vi "windows_folder_paths.vi"(8 "error in (no error)":errorcluster, 9 "Create Folder if not found? (F)":bool, 10 "Return non-default path?":enum32{"current path", "default path"}(ring), 11 "Folder Role":i32(ring)) -> (0 "error out":errorcluster {"code" format="%.0x"}, 1 "Description":string, 3 "System Folder Path":path)   [LabVIEW 2015]
doc: "This VI calls a Windows API function to retrieve the path of Windows System Folders that may vary with different installations of the operating system."
uses:
  shell32.dll
panel:
  # "These are CSIDL (constant special item ID list)\ncodes from the Windows API"
  # "The current folder may differ from the \ndefault if the user moved it or renamed it."
  # "Note:  CSIDL values are defined in Windows header file shlobj.h. \nFor a list of CSIDL constants, search Microsoft's web site for \"CSIDL\".\n\nThe function and constants used in this VI are supported on Win2000,\nWinXP, and Vista."
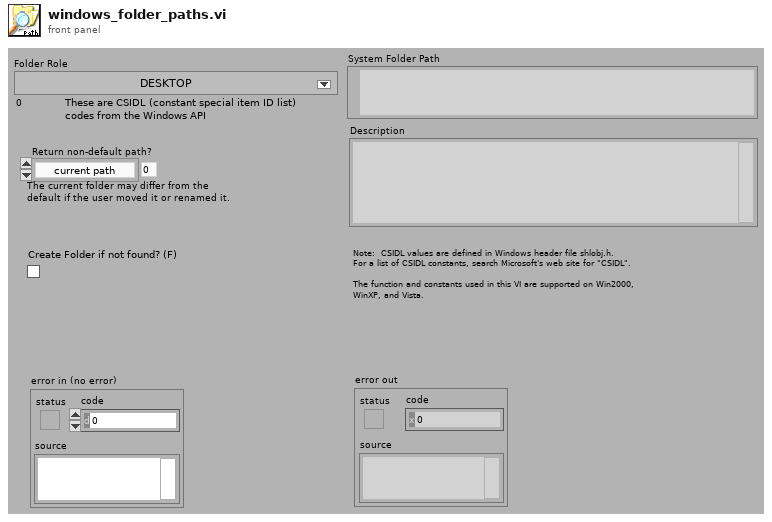
[diagram p1: front panel]
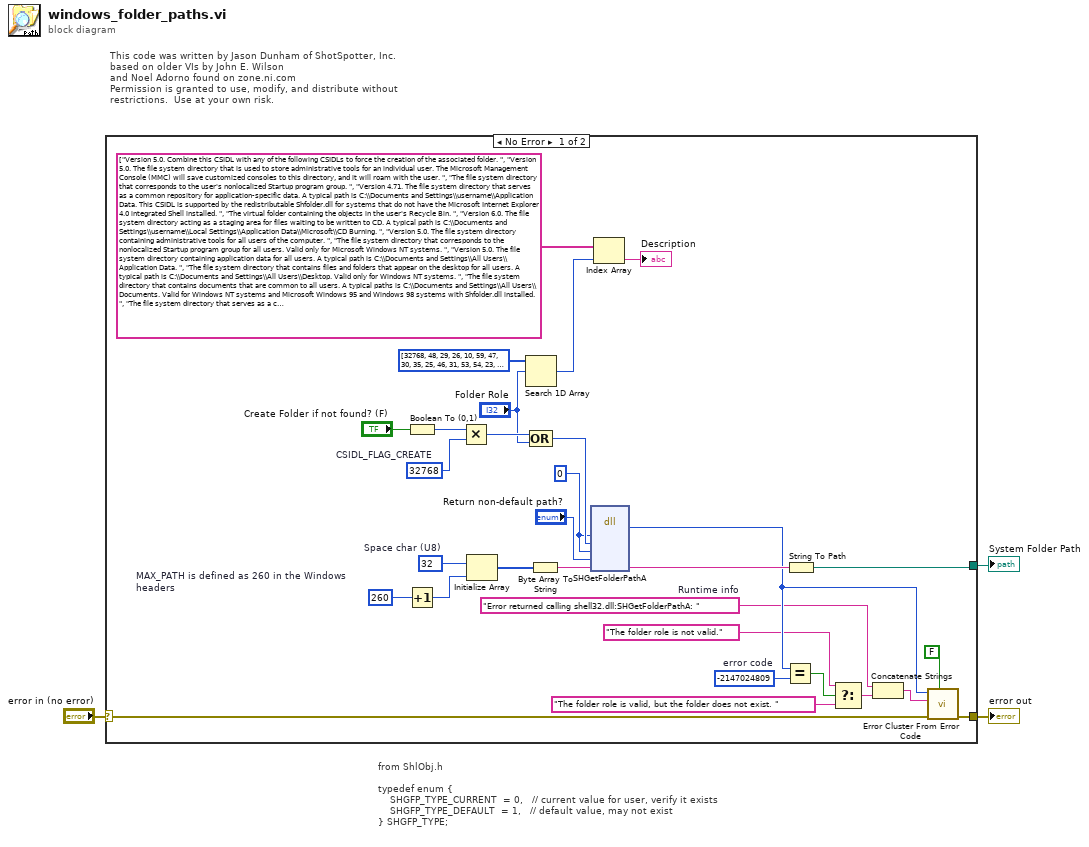
[diagram p0: block diagram]
diagram:
  # "This code was written by Jason Dunham of ShotSpotter, Inc.\nbased on older VIs by John E. Wilson\nand Noel Adorno found on zone.ni.com\nPermission is granted to use, modify, and distribute without \nrestrictions.  Use at your own risk."
  # "from ShlObj.h \n\ntypedef enum {\n    SHGFP_TYPE_CURRENT  = 0,   // current value for user, verify it exists\n    SHGFP_TYPE_DEFAULT  = 1,   // default value, may not exist\n} SHGFP_TYPE;"
  n1 = case shown="No Error" "error in (no error)" {
    selector: "error in (no error)" -> [w15 w34]
    tunnel: [w17 _] -> w3
    tunnel: [w14 w34] -> w1
    frame No Error {
      w21 = u8 32  # Space char (U8)
      w6 = "Error returned calling shell32.dll:SHGetFolderPathA: "  # Runtime info
      w11 = -2147024809  # error code
      w23 = 260  # MAX_PATH is defined as 260 in the Windows headers
      w25 = 32768  # CSIDL_FLAG_CREATE
      w4 = 0 ("hwind")
      n2 = Boolean To (0,1)(Boolean="Create Folder if not found? (F)") -> (0, 1=w26:i16)
      n3 = Increment(x=w23) -> (x+1=w22:i32)
      n4 = Multiply(x=w26, y=w25) -> (x*y=w24:i32)
      n5 = Initialize Array(w21, w22) -> (w20:u8[])
      n6 = Search 1D Array(1D array=u32[] [32768, 48, 29, 26, 10, 59, 47, 30, 35, 25, 46, 31, 53, 54, 23, 22, 24, 45, 55, 61, 49, 3, 33, 0, 16, 17, 6, 16384, 20, 34, 1, 32, 28, 12, 13, 39, 14, 19, 18, 5, 69, 63, 4, 27, 40, 38, 43, 2, 8, 56, 64, 65, 66, 67, 9, 11, 7, 37, 21, 36] ("Array 2"), element="Folder Role") -> (index of element=w30:i32)  [unwired: 1 out]
      n7 = Compound Arithmetic op=OR(w24, "Folder Role") -> (w16:i32)
      n8 = Byte Array To String(unsigned byte array=w20) -> (string=w19:string)
      n9 = dll-call lib="shell32.dll" fn="SHGetFolderPathA"("hwind"=w4, "nFolder"=w16, "htoken"=w4, "flags"="Return non-default path?", "path"=w19) -> ("return value"=w12:i32, "path"=w32:string)  [unwired: 6 in, 3 out]
      n10 = Index Array(array=string[] ["Version 5.0. Combine this CSIDL with any of the following CSIDLs to force the creation of the associated folder. ", "Version 5.0. The file system directory that is used to store administrative tools for an individual user. The Microsoft Management Console (MMC) will save customized consoles to this directory, and it will roam with the user. ", "The file system directory that corresponds to the user's nonlocalized Startup program group. ", "Version 4.71. The file system directory that serves as a common repository for application-specific data. A typical path is C:\\Documents and Settings\\username\\Application Data. This CSIDL is supported by the redistributable Shfolder.dll for systems that do not have the Microsoft Internet Explorer 4.0 integrated Shell installed. ", "The virtual folder containing the objects in the user's Recycle Bin. ", "Version 6.0. The file system directory acting as a staging area for files waiting to be written to CD. A typical path is C:\\Documents and Settings\\username\\Local Settings\\Application Data\\Microsoft\\CD Burning. ", "Version 5.0. The file system directory containing administrative tools for all users of the computer. ", "The file system directory that corresponds to the nonlocalized Startup program group for all users. Valid only for Microsoft Windows NT systems. ", "Version 5.0. The file system directory containing application data for all users. A typical path is C:\\Documents and Settings\\All Users\\Application Data. ", "The file system directory that contains files and folders that appear on the desktop for all users. A typical path is C:\\Documents and Settings\\All Users\\Desktop. Valid only for Windows NT systems. ", "The file system directory that contains documents that are common to all users. A typical paths is C:\\Documents and Settings\\All Users\\Documents. Valid for Windows NT systems and Microsoft Windows 95 and Windows 98 systems with Shfolder.dll installed. ", "The file system directory that serves as a common repository for favorite items common to all users. Valid only for Windows NT systems. ", "Version 6.0. The file system directory that serves as a repository for music files common to all users. A typical path is C:\\Documents and Settings\\All Users\\Documents\\My Music. ", "Version 6.0. The file system directory that serves as a repository for image files common to all users. A typical path is C:\\Documents and Settings\\All Users\\Documents\\My Pictures. ", "The file system directory that contains the directories for the common program groups that appear on the Start menu for all users. A typical path is C:\\Documents and Settings\\All Users\\Start Menu\\Programs. Valid only for Windows NT systems. ", "The file system directory that contains the programs and folders that appear on the Start menu for all users. A typical path is C:\\Documents and Settings\\All Users\\Start Menu. Valid only for Windows NT systems. ", "The file system directory that contains the programs that appear in the Startup folder for all users. A typical path is C:\\Documents and Settings\\All Users\\Start Menu\\Programs\\Startup. Valid only for Windows NT systems. ", "The file system directory that contains the templates that are available to all users. A typical path is C:\\Documents and Settings\\All Users\\Templates. Valid only for Windows NT systems. ", "Version 6.0. The file system directory that serves as a repository for video files common to all users. A typical path is C:\\Documents and Settings\\All Users\\Documents\\My Videos. ", "The folder representing other machines in your workgroup. ", "The virtual folder representing Network Connections, containing network and dial-up connections. ", "The virtual folder containing icons for the Control Panel applications. ", "The file system directory that serves as a common repository for Internet cookies. A typical path is C:\\Documents and Settings\\username\\Cookies. ", "The virtual folder representing the Windows desktop, the root of the namespace. ", "The file system directory used to physically store file objects on the desktop (not to be confused with the desktop folder itself). A typical path is C:\\Documents and Settings\\username\\Desktop. ", "The virtual folder representing My Computer, containing everything on the local computer: storage devices, printers, and Control Panel. The folder may also contain mapped network drives. ", "The file system directory that serves as a common repository for the user's favorite items. A typical path is C:\\Documents and Settings\\username\\Favorites. ", "Combine with another CSIDL constant, except for CSIDL_FLAG_CREATE, to return an unverified folder pathwith no attempt to create or initialize the folder. ", "A virtual folder containing fonts. A typical path is C:\\Windows\\Fonts. ", "The file system directory that serves as a common repository for Internet history items. ", "A viritual folder for Internet Explorer (icon on desktop). ", "Version 4.72. The file system directory that serves as a common repository for temporary Internet files. A typical path is C:\\Documents and Settings\\username\\Local Settings\\Temporary Internet Files. ", "Version 5.0. The file system directory that serves as a data repository for local (nonroaming) applications. A typical path is C:\\Documents and Settings\\username\\Local Settings\\Application Data. ", "Version 6.0. The virtual folder representing the My Documents desktop item. ", "The file system directory that serves as a common repository for music files. A typical path is C:\\Documents and Settings\\User\\My Documents\\My Music. ", "Version 5.0. The file system directory that serves as a common repository for image files. A typical path is C:\\Documents and Settings\\username\\My Documents\\My Pictures. ", "Version 6.0. The file system directory that serves as a common repository for video files. A typical path is C:\\Documents and Settings\\username\\My Documents\\My Videos. ", "A file system directory containing the link objects that may exist in the My Network Places virtual folder. It is not the same as CSIDL_NETWORK, which represents the network namespace root. A typical path is C:\\Documents and Settings\\username\\NetHood. ", "A virtual folder representing Network Neighborhood, the root of the network namespace hierarchy. ", "Version 6.0. The virtual folder representing the My Documents desktop item. This is equivalent to CSIDL_MYDOCUMENTS. _________ Previous to Version 6.0. The file system directory used to physically store a user's common repository of documents. A typical path is C:\\Documents and Settings\\username\\My Documents. This should be distinguished from the virtual My Documents folder in the namespace. To access that virtual folder, use SHGetFolderLocation, which returns the ITEMIDLIST for the virtual location, or refer to the technique described in Managing the File System.", "Note  This documentation is preliminary and is subject to change._______  Windows Vista and later. The virtual folder used to store photo albums, typically username\\My Pictures\\Photo Albums. ", "Note  This documentation is preliminary and is subject to change.  _______  Windows Vista and later. The virtual folder used to store play albums, typically username\\My Music\\Playlists. ", "The virtual folder containing installed printers. ", "The file system directory that contains the link objects that can exist in the Printers virtual folder. A typical path is C:\\Documents and Settings\\username\\PrintHood. ", "Version 5.0. The user's profile folder. A typical path is C:\\Documents and Settings\\username. Applications should not create files or folders at this level; they should put their data under the locations referred to by CSIDL_APPDATA or CSIDL_LOCAL_APPDATA. ", "Version 5.0. The Program Files folder. A typical path is C:\\Program Files. ", "Version 5.0. A folder for components that are shared across applications. A typical path is C:\\Program Files\\Common. Valid only for Windows NT, Windows 2000, and Windows XP systems. Not valid for Windows Millennium Edition (Windows Me). ", "The file system directory that contains the user's program groups (which are themselves file system directories). A typical path is C:\\Documents and Settings\\username\\Start Menu\\Programs. ", "The file system directory that contains shortcuts to the user's most recently used documents. A typical path is C:\\Documents and Settings\\username\\My Recent Documents. To create a shortcut in this folder, use SHAddToRecentDocs. In addition to creating the shortcut, this function updates the Shell's list of recent documents and adds the shortcut to the My Recent Documents submenu of the Start menu. ", "Note  This documentation is preliminary and is subject to change. _________ Windows Vista and later. The file system directory that contains resource data. A typical path is C:\\Windows\\Resources. ", "Note  This documentation is preliminary and is subject to change. ___________Windows Vista and later. The file system directory that contains sample music. A typical path is C:\\Documents and Settings\\username\\My Documents\\My Music\\Sample Music. ", "Note  This documentation is preliminary and is subject to change. __________Windows Vista and later. The file system directory that contains sample playlists. A typical path is C:\\Documents and Settings\\username\\My Documents\\My Music\\Sample Playlists. ", "Note  This documentation is preliminary and is subject to change. ________ Windows Vista and later. The file system directory that contains sample pictures. A typical path is C:\\Documents and Settings\\username\\My Documents\\My Pictures\\Sample Pictures. ", "Note  This documentation is preliminary and is subject to change. ________  Windows Vista and later. The file system directory that contains sample videos. A typical path is C:\\Documents and Settings\\username\\My Documents\\My Videos\\Sample Videos. ", "The file system directory that contains Send To menu items. A typical path is C:\\Documents and Settings\\username\\SendTo. ", "The file system directory containing Start menu items. A typical path is C:\\Documents and Settings\\username\\Start Menu. ", "The file system directory that corresponds to the user's Startup program group. The system starts these programs whenever any user logs onto Windows NT or starts Windows 95. A typical path is C:\\Documents and Settings\\username\\Start Menu\\Programs\\Startup. ", "Version 5.0. The Windows System folder. A typical path is C:\\Windows\\System32. ", "The file system directory that serves as a common repository for document templates. A typical path is C:\\Documents and Settings\\username\\Templates. ", "Version 5.0. The Windows directory or SYSROOT. This corresponds to the %windir% or %SYSTEMROOT% environment variables. A typical path is C:\\Windows."] ("Array"), index=w30) -> (element=→"Description":string)
      n11 = Equal?(x=w12, y=w11) -> (x = y?=w10:bool)
      n12 = String To Path(string=w32) -> (path=w17:path)
      n13 = Select(t="The folder role is not valid.", s=w10, f="The folder role is valid, but the folder does not exist. ") -> (s? t:f=w7:string)
      n14 = Concatenate Strings(w6, w7) -> (w5:string)
      n15 = call <vilib>:"Error Cluster From Error Code.vi"("show call chain? (False)"=FALSE, "error in (no error)"=w15, "error message (\"\")"=w5, "error code (0)"=w12) -> ("error out"=w14:errorcluster)  [unwired: 5 out]
    }
    frame Error {
    }
  }
  "error out" <- w1
  "System Folder Path" <- w3
